vi "terminate_main.vi"(8 "error in (no error)":errorcluster) -> (0 "error out":errorcluster)   [LabVIEW 2010]
uses:
  components/ExperimentController/GenericExperimentController/GenericExperimentController/GenericExperimentController.lvclass
  components/ImagingMode/GenericImagingMode/GenericImagingMode/GenericImagingMode.lvclass
  components/ScanHead/GenericScanHead/GenericScanHead/GenericScanHead.lvclass
  components/DAQ/GenericDAQ/GenericDAQ/GenericDAQ.lvclass
  components/ImageAssembler/GenericImageAssembler/GenericImageAssembler/GenericImageAssembler.lvclass
  components/DataCollection/GenericDataCollection/GenericDataCollection/GenericDataCollection.lvclass
  components/Display/GenericDisplay/GenericDisplay/GenericDisplay.lvclass
  components/Stage/GenericStage/GenericStage/GenericStage.lvclass
  components/Stimulator/GenericStimulator/GenericStimulator/GenericStimulator.lvclass
  components/Analyser/GenericAnalyser/GenericAnalyser/GenericAnalyser.lvclass
  components/Instrument/GenericInstrument/GenericInstrument/GenericInstrument.lvclass
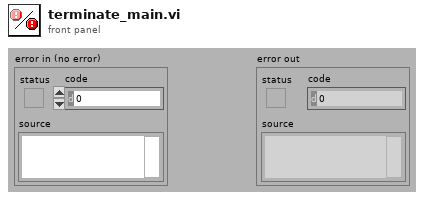
[diagram p1: front panel]
types:
  T1 = enum8{"Enabled", "Disabled", "Disabled and Grayed Out"}
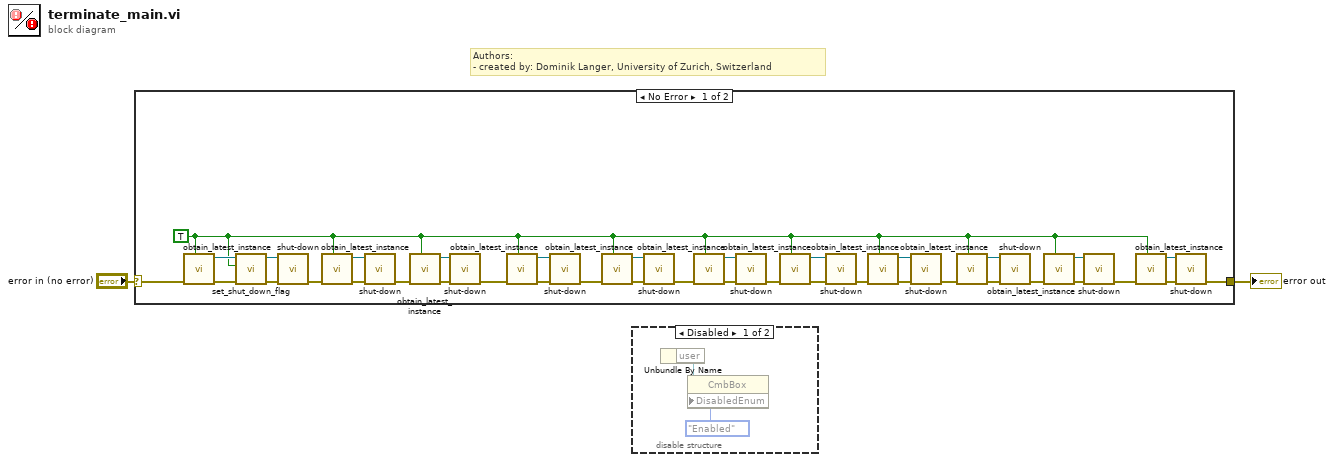
[diagram p0: block diagram]
diagram:
  # "Authors: \n- created by: Dominik Langer, University of Zurich, Switzerland"
  n1 = case shown="No Error" "error in (no error)" {
    selector: "error in (no error)" -> [w4 w40]
    tunnel: [w3 w40] -> w2
    frame No Error {
      w5 = TRUE
      n2 = call "obtain_latest_instance.vi"("quick, but maybe outdated?"=w5, "error in (no error)"=w4) -> ("error out"=w9:errorcluster, "GenericExperimentController out"=w7:refnum<class "GenericExperimentController.lvclass">)  [unwired: 8 out]
      n3 = call-dynamic "set_shut_down_flag.vi"("error in (no error)"=w9, "shut down?"=w5, "GenericPlugin in"=w7) -> ("error out"=w8:errorcluster, "GenericPlugin out"=w6:refnum<class "GenericExperimentController.lvclass">)  [unwired: 7 out]
      n4 = call-dynamic "shut-down.vi"("error in (no error)"=w8, "GenericToplevelComponent in"=w6) -> ("error out"=w30:errorcluster)  [unwired: 9 out]
      n5 = call "obtain_latest_instance.vi"("quick, but maybe outdated?"=w5, "error in (no error)"=w30) -> ("error out"=w23:errorcluster, "GenericScanMode out"=w22:refnum<class "GenericImagingMode.lvclass">)  [unwired: 8 out]
      n6 = call-dynamic "shut-down.vi"("error in (no error)"=w23, "GenericToplevelComponent in"=w22) -> ("error out"=w21:errorcluster)  [unwired: 9 out]
      n7 = call "obtain_latest_instance.vi"("quick, but maybe outdated?"=w5, "error in (no error)"=w21) -> ("error out"=w26:errorcluster, "GenericScanHead out"=w25:refnum<class "GenericScanHead.lvclass">)  [unwired: 8 out]
      n8 = call-dynamic "shut-down.vi"("error in (no error)"=w26, "GenericToplevelComponent in"=w25) -> ("error out"=w24:errorcluster)  [unwired: 9 out]
      n9 = call "obtain_latest_instance.vi"("quick, but maybe outdated?"=w5, "error in (no error)"=w24) -> ("error out"=w39:errorcluster, "GenericDAQ out"=w38:refnum<class "GenericDAQ.lvclass">)  [unwired: 8 out]
      n10 = call-dynamic "shut-down.vi"("error in (no error)"=w39, "GenericToplevelComponent in"=w38) -> ("error out"=w37:errorcluster)  [unwired: 9 out]
      n11 = call "obtain_latest_instance.vi"("quick, but maybe outdated?"=w5, "error in (no error)"=w37) -> ("error out"=w29:errorcluster, "GenericImageAssembler out"=w28:refnum<class "GenericImageAssembler.lvclass">)  [unwired: 8 out]
      n12 = call-dynamic "shut-down.vi"("error in (no error)"=w29, "GenericToplevelComponent in"=w28) -> ("error out"=w27:errorcluster)  [unwired: 9 out]
      n13 = call "obtain_latest_instance.vi"("quick, but maybe outdated?"=w5, "error in (no error)"=w27) -> ("error out"=w36:errorcluster, "GenericDataCollection out"=w35:refnum<class "GenericDataCollection.lvclass">)  [unwired: 8 out]
      n14 = call-dynamic "shut-down.vi"("error in (no error)"=w36, "GenericToplevelComponent in"=w35) -> ("error out"=w34:errorcluster)  [unwired: 9 out]
      n15 = call "obtain_latest_instance.vi"("quick, but maybe outdated?"=w5, "error in (no error)"=w34) -> ("error out"=w32:errorcluster, "GenericDisplay out"=w33:refnum<class "GenericDisplay.lvclass">)  [unwired: 8 out]
      n16 = call-dynamic "shut-down.vi"("error in (no error)"=w32, "GenericToplevelComponent in"=w33) -> ("error out"=w31:errorcluster)  [unwired: 9 out]
      n17 = call "obtain_latest_instance.vi"("quick, but maybe outdated?"=w5, "error in (no error)"=w31) -> ("error out"=w20:errorcluster, "GenericStage out"=w19:refnum<class "GenericStage.lvclass">)  [unwired: 8 out]
      n18 = call-dynamic "shut-down.vi"("error in (no error)"=w20, "GenericToplevelComponent in"=w19) -> ("error out"=w18:errorcluster)  [unwired: 9 out]
      n19 = call "obtain_latest_instance.vi"("quick, but maybe outdated?"=w5, "error in (no error)"=w18) -> ("error out"=w17:errorcluster, "GenericStimulator out"=w16:refnum<class "GenericStimulator.lvclass">)  [unwired: 8 out]
      n20 = call-dynamic "shut-down.vi"("error in (no error)"=w17, "GenericToplevelComponent in"=w16) -> ("error out"=w15:errorcluster)  [unwired: 9 out]
      n21 = call "obtain_latest_instance.vi"("quick, but maybe outdated?"=w5, "error in (no error)"=w15) -> ("error out"=w12:errorcluster, "GeneralAnalyser out"=w10:refnum<class "GenericAnalyser.lvclass">)  [unwired: 8 in]
      n22 = call-dynamic "shut-down.vi"("error in (no error)"=w12, "GenericToplevelComponent in"=w10) -> ("error out"=w11:errorcluster)  [unwired: 8 in, 1 out]
      n23 = call "obtain_latest_instance.vi"("quick, but maybe outdated?"=w5, "error in (no error)"=w11) -> ("error out"=w14:errorcluster, "microscope"=w13:refnum<class "GenericInstrument.lvclass">)  [unwired: 8 in]
      n24 = call-dynamic "shut-down.vi"("error in (no error)"=w14, "GenericToplevelComponent in"=w13) -> ("error out"=w3:errorcluster)  [unwired: 8 in, 1 out]
    }
    frame Error {
    }
  }
  "error out" <- w2
  n25 = disable-structure shown="Disabled" {
    frame Disabled {
      n26 = Unbundle By Name() -> ("user"=w42:refnum<vi>)  [unwired: 1 in]
      n27 = property class="CmbBox"(reference=w42, "DisabledEnum"=T1."Enabled" ("Disabled")) -> ()  [unwired: 1 in, 2 out]
    }
    frame Enabled {
    }
  }
